vi "Flash Firmware.vi"(8 "error in":errorcluster, 11 "Spark Reference In":T1) -> (3 "Spark Reference Out":T1)   [LabVIEW 2013, in "Spark API.lvlib"]
uses:
  Spark API.lvlib
  Controls/Spark Reference.ctl
  <vilib>/httpClient/ClientHandle.ctl
  Controls/Device Query JSON.ctl
  <vilib>/httpClient/LabVIEWHTTPClient.lvlib
panel:
  out "error out":errorcluster
  in  "Path to Code":path=path "/iMac SSD/Users/fred/Documents/Git Repositories/Spark API/code.cpp"
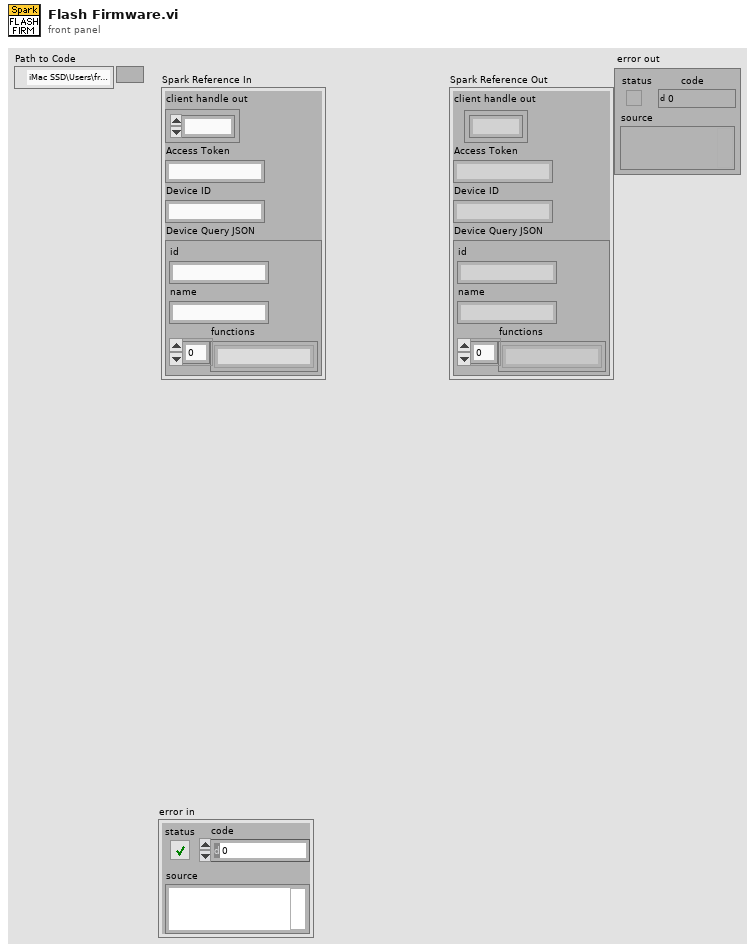
[diagram p1: front panel]
types:
  T1 = typedef "Spark API.lvlib/Spark Reference.ctl" = cluster{"client handle out":T2, "Access Token":string, "Device ID":string, "Device Query JSON":T3}
  T2 = typedef "LabVIEWHTTPClient.lvlib/ClientHandle.ctl" = refnum<k1>
  T3 = typedef "Spark API.lvlib/Device Query JSON.ctl" = cluster{"id":string, "name":string, "functions":string[]}
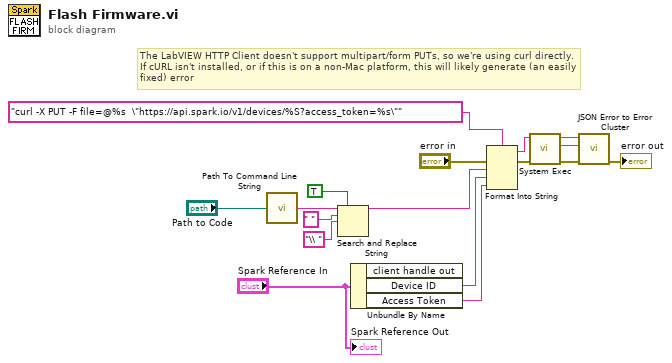
[diagram p0: block diagram]
diagram:
  # "The LabVIEW HTTP Client doesn't support multipart/form PUTs, so we're using curl directly. If cURL isn't installed, or if this is on a non-Mac platform, this will likely generate (an easily fixed) error"
  n1 = call <vilib>:"Path To Command Line String.vi"("path"="Path to Code") -> ("string"=w7:string)
  n2 = Search and Replace String(replace all?=TRUE ("replace all? (F)"), input string=w7, search string=" ", replace string="\\ " ("replace string (\"\")")) -> (result string=w8:string)  [unwired: 4 in, 3 out]
  n3 = Unbundle By Name("Spark Reference In") -> ("Device ID"=w12:string, "Access Token"=w14:string)  [unwired: 1 out]
  n4 = Format Into String(format string="curl -X PUT -F file=@%s  \"https://api.spark.io/v1/devices/%S?access_token=%s\"" ("url"), error in="error in", w8, w12, w14) -> (resulting string=w11:string, error out=w10:errorcluster)  [unwired: 1 in]
  n5 = call <vilib>:"System Exec.vi"("error in (no error)"=w10, "command line"=w11) -> ("error out"=w9:errorcluster, "standard error"=w2:string, "standard output"=w1:string)  [unwired: 6 in, 1 out]
  n6 = call "JSON Error to Error Cluster.vi"("error in (no error)"=w9, "headers"=w2, "JSON string"=w1) -> ("error out"=→"error out":errorcluster)  [unwired: 8 in]
  "Spark Reference Out" <- "Spark Reference In"
